vi "RxDataDeal.vi"(7 "dataByteNumb":dbl, 8 "error in (no error)":errorcluster caption="错误输入（无错误）", 9 "freqDiv":dbl, 10 "udp_data_rr0":dbl[](array[numeric]), 11 "Path":path) -> (0 "error out":errorcluster caption="错误输出", 2 "rxdataQ":dbl[](array[numeric]), 3 "rxdataI":dbl[](array[numeric]))   [LabVIEW 2015]
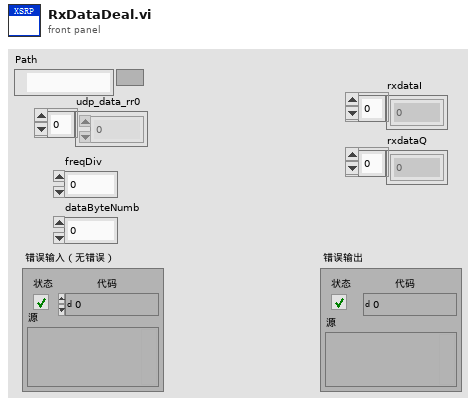
[diagram p1: front panel]
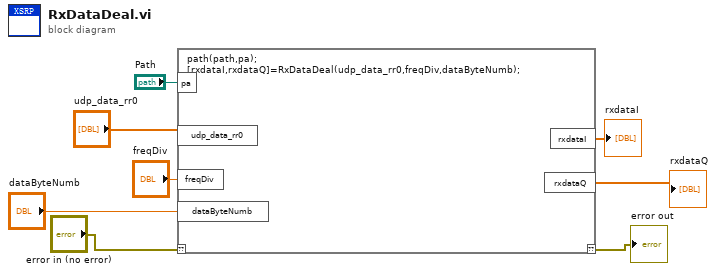
[diagram p0: block diagram]
diagram:
  n1 = script code="path(path,pa);\n[rxdataI,rxdataQ]=RxDataDeal(udp_data_rr0,freqDiv,dataByteNumb);"("??"="error in (no error)", "pa"="Path", "udp_data_rr0"="udp_data_rr0", "freqDiv"="freqDiv", "dataByteNumb"="dataByteNumb") -> ("??"=→"error out":errorcluster, "rxdataI"=→"rxdataI":dbl[], "rxdataQ"=→"rxdataQ":dbl[])
